vi "Write_Ch_data_file.vi"(4 "Append last row only":bool, 5 "Header string":string, 7 "exists?":bool, 8 "Write offset fr file end":i32, 9 "Channel Values":string[][](array[string]), 10 "Channel names":string[](array[string]), 11 "Filename":path) -> ()   [LabVIEW 2020]
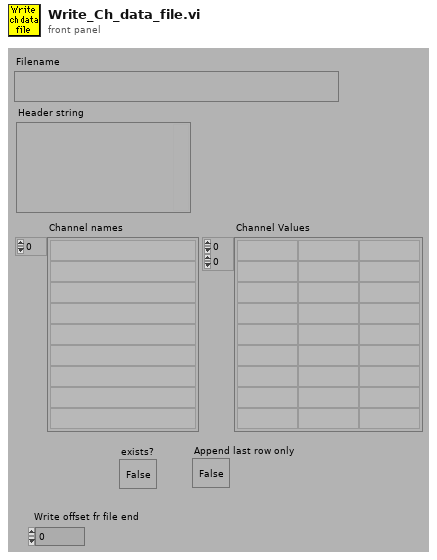
[diagram p1: front panel]
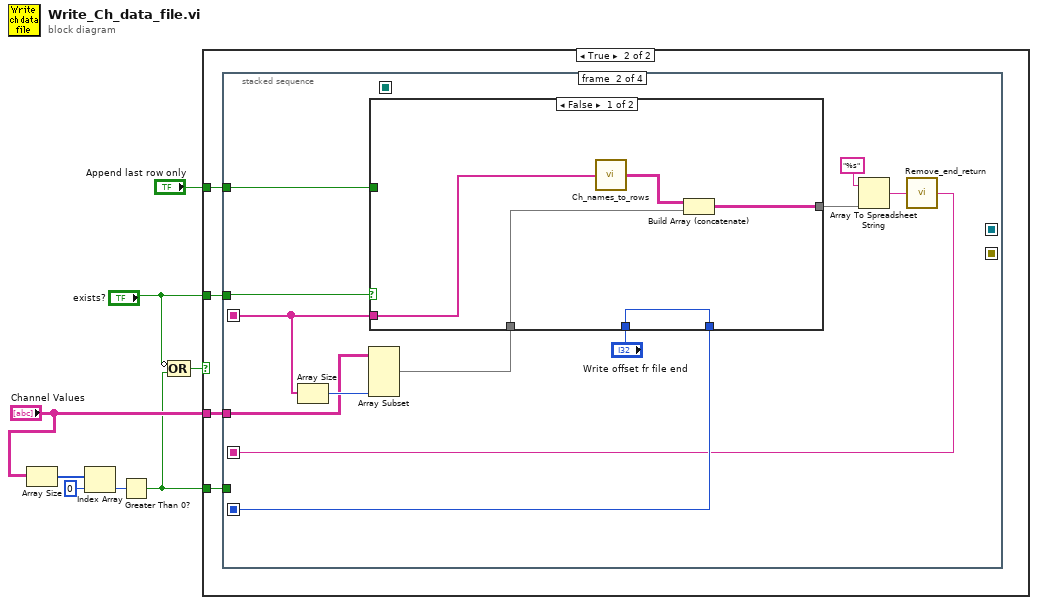
[diagram p0: block diagram]
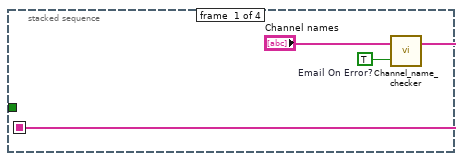
[diagram p3: hidden frame]
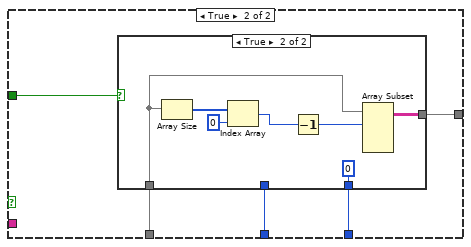
[diagram p4: hidden frame]
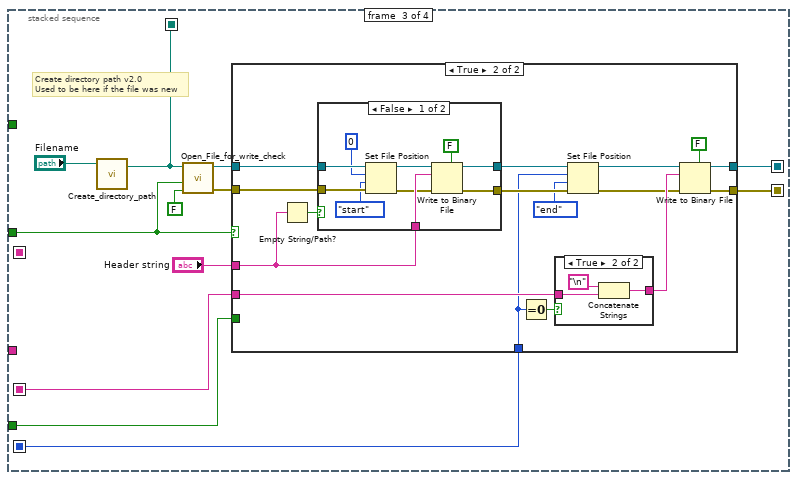
[diagram p6: hidden frame]
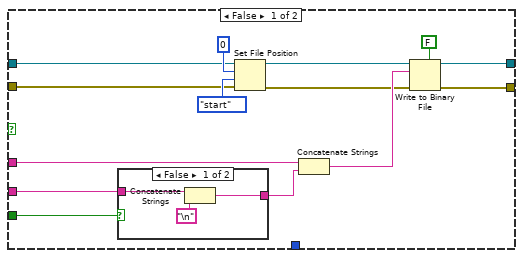
[diagram p7: hidden frame]
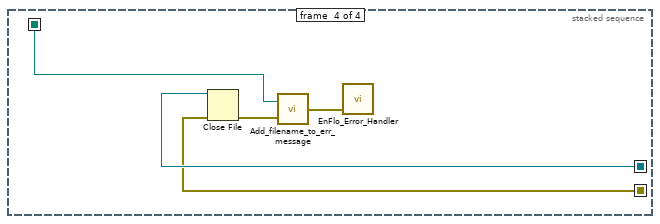
[diagram p11: hidden frame]
diagram:
  n1 = Array Size(array="Channel Values") -> (size(s)=w5:i32[])
  n2 = Index Array(array=w5, index=0 ("Index")) -> (element=w4:i32)
  n3 = Greater Than 0?(x=w4) -> (x > 0?=w1:bool)
  n4 = Compound Arithmetic op=OR(invert "exists?", w1) -> (w2:bool)
  n5 = case shown="True" w2 {
    tunnel: "exists?" -> [_ w12]
    tunnel: "Append last row only" -> [_ w11]
    tunnel: "Channel Values" -> [_ w10]
    tunnel: w1 -> [_ w9]
    frame False {
    }
    frame True {
      n6 = stacked-sequence {
        seq-local: [_ w21 _ _] -> [_ _ w58 _]
        seq-local: [_ w24 _ _] -> [_ _ w55 _]
        seq-local: [_ _ w56 _] -> [_ _ _ w113]
        seq-local: [_ _ w54 _] -> [_ _ _ w112]
        seq-local: [w15 _ _ _] -> [_ w17 _ _]
        seq-local: [_ _ w48 _] -> [_ _ _ w110]
        tunnel: w12 -> [_ w23 w50 _]
        tunnel: w11 -> [_ w25 _ _]
        tunnel: w10 -> [_ w18 _ _]
        tunnel: w9 -> [_ _ w47 _]
        frame #0 {
          w13 = TRUE  # Email On Error?
          n7 = call "Channel_name_checker.vi"("Email On Error?"=w13, "Channel names"="Channel names") -> ("Channel names Out"=w15:string[])  [unwired: 1 out]
        }
        frame #1 {
          n8 = Array Size(array=w17) -> (size(s)=w19:i32)
          n9 = Array Subset(array=w18, length (col)=w19) -> (w16:string[][])  [unwired: 3 in]
          n10 = case shown="False" w23 {
            tunnel: w17 -> [w29 _]
            tunnel: [w32 w34] -> w26
            tunnel: w25 -> [_ w37]
            tunnel: [w31 w36] -> w24
            tunnel: "Write offset fr file end" -> [w31 w35]
            tunnel: w16 -> [w28 w33]
            frame False {
              n11 = call "Ch_names_to_rows.vi"("Channel Names"=w29) -> ("3 Row names"=w30:string[][])
              n12 = Build Array (concatenate)(w30, w28) -> (w32:string[][])
            }
            frame True {
              n13 = case shown="True" w37 {
                tunnel: w33 -> [w39 w42]
                tunnel: [w39 w41] -> w34
                tunnel: [w38 0 ("Write offset fr file end")] -> w36
                tunnel: w35 -> [w38 _]
                frame False {
                }
                frame True {
                  n14 = Array Size(array=w42) -> (size(s)=w45:i32[])
                  n15 = Index Array(array=w45, index=0) -> (element=w43:i32)
                  n16 = Decrement(x=w43) -> (x-1=w44:i32)
                  n17 = Array Subset(array=w42, index (row)=w44) -> (w41:string[][])  [unwired: 3 in]
                }
              }
            }
          }
          n18 = Array To Spreadsheet String(array=w26, 3:"%s" ("format string")) -> (spreadsheet string=w22:string)  [unwired: 1 out]
          n19 = call "Remove_end_return.vi"("Input string"=w22) -> ("Output string"=w21:string)
        }
        frame #2 {
          # "Create directory path v2.0\nUsed to be here if the file was new"
          n20 = call "Create_directory_path.vi"("Path name"="Filename") -> ("Path name Out"=w48:path)  [unwired: 2 in, 1 out]
          n21 = call "Open_File_for_write_check.vi"("advisory dialog? (display:T)"=FALSE, "append to file? (new file:F)"=w50, "file path"=w48) -> ("error out"=w53:errorcluster, "refnum"=w51:refnum<file>)  [unwired: 7 out]
          n22 = case shown="True" w50 {
            tunnel: w55 -> [_ w85]
            tunnel: w58 -> [w59 w88]
            tunnel: [w70 w90] -> w54
            tunnel: "Header string" -> [w69 w78]
            tunnel: [w67 w89] -> w56
            tunnel: w51 -> [w66 w83]
            tunnel: w53 -> [w65 w84]
            tunnel: w47 -> [w61 _]
            frame False {
              n23 = case shown="False" w61 {
                tunnel: [w73 w76] -> w60
                tunnel: w59 -> [w74 w76]
                frame False {
                  n24 = Concatenate Strings(w74, "\n") -> (w73:string)
                }
                frame True {
                }
              }
              n25 = Set File Position(offset (in bytes) (0)=0 ("pos offset (0)"), refnum=w66, from (0:start)=enum16{"start", "end", "current"}."start" ("pos mode (0:2)"), error in=w65) -> (refnum out=w64:refnum<file>, error out=w63:errorcluster)
              n26 = Concatenate Strings(w69, w60) -> (w68:string)
              n27 = Write to Binary File(file (use dialog)=w64, data=w68, error in=w63, 5:FALSE ("prepend array or string size? (T)")) -> (refnum out=w67:refnum<file>, error out=w70:errorcluster)  [unwired: 3 out]
            }
            frame True {
              n28 = Empty String/Path?(string/path=w78) -> (empty?=w77:bool)
              n29 = case shown="False" w77 {
                tunnel: w83 -> [w106 w108]
                tunnel: w84 -> [w105 w107]
                tunnel: [w102 w108] -> w92
                tunnel: [w101 w107] -> w91
                tunnel: w78 -> [w100 _]
                frame False {
                  n30 = Set File Position(offset (in bytes) (0)=0 ("pos offset (0)"), refnum=w106, from (0:start)=enum16{"start", "end", "current"}."start" ("pos mode (0:2)"), error in=w105) -> (refnum out=w99:refnum<file>, error out=w98:errorcluster)
                  n31 = Write to Binary File ("Write File")(file (use dialog)=w99, data=w100, error in=w98, 5:FALSE ("prepend array or string size? (T)")) -> (refnum out=w102:refnum<file>, error out=w101:errorcluster)  [unwired: 3 out]
                }
                frame True {
                }
              }
              n32 = Equal To 0?(x=w85) -> (x = 0?=w86:bool)
              n33 = case shown="True" w86 {
                tunnel: w88 -> [w93 w96]
                tunnel: [w93 w95] -> w87
                frame False {
                }
                frame True {
                  n34 = Concatenate Strings("\n", w96) -> (w95:string)
                }
              }
              n35 = Set File Position(offset (in bytes) (0)=w85, refnum=w92, from (0:start)=enum16{"start", "end", "current"}."end" ("pos mode (0:2)"), error in=w91) -> (refnum out=w81:refnum<file>, error out=w80:errorcluster)
              n36 = Write to Binary File(file (use dialog)=w81, data=w87, error in=w80, 5:FALSE ("prepend array or string size? (T)")) -> (refnum out=w89:refnum<file>, error out=w90:errorcluster)  [unwired: 3 out]
            }
          }
        }
        frame #3 {
          n37 = Close File(refnum=w113, error in=w112) -> (error out=w111:errorcluster)  [unwired: 1 out]
          n38 = call "Add_filename_to_err_message.vi"("error in (no error)"=w111, "Path"=w110) -> ("error out"=w109:errorcluster)
          n39 = call "EnFlo_Error_Handler.vi"("error in (no error)"=w109) -> ()  [unwired: 2 in, 3 out]
        }
      }
    }
  }
